vi "Set status to Idle.vi"(10 "Next state queue data":T1, 11 "UI queue":refnum<queue>) -> ()   [LabVIEW 2013]
uses:
  Typedefs/Next state queue data.ctl
  Typedefs/Start-Stop Enum.ctl
  Typedefs/Top level VI states.ctl
  Queue/Message Queue/Typedefs/Message Cluster.ctl
  Global Variables/General Globals.vi
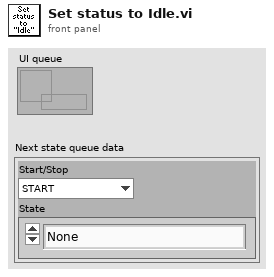
[diagram p1: front panel]
types:
  T1 = typedef "Next state queue data.ctl" = cluster{"Start/Stop":T2, "State":T3}
  T2 = typedef "Start-Stop Enum.ctl" = enum16{"START", "STOP"}
  T3 = typedef "Top level VI states.ctl" = enum16{"None", "Initialise UI", "<STACK PROTOCOL STATES>", "AOL Zstack-START", "AOL Zstack-STOP", "Motor Zstack-START", "Motor Zstack-STOP", "<ACQUISITION PROTOCOL STATES> ", "Functional Acquisition-START", "Functional Acquisition-STOP", "Single Plane Acquisition-START", "Single Plane Acquisition-STOP", "Volume Acquisition-START", "Volume Acquisition-STOP", "<LIVE IMAGING PROTOCOL STATES>", "Live Imaging-START", "Live Imaging-STOP", "Live Plane Imaging-START", "Live Plane Imaging-STOP", "Live Volume Imaging-START", "Live Volume Imaging-STOP", "EXIT"}
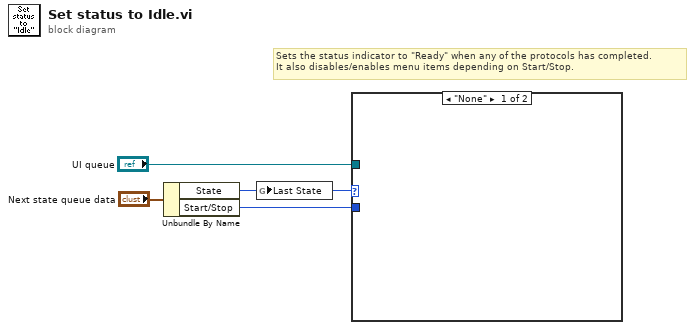
[diagram p0: block diagram]
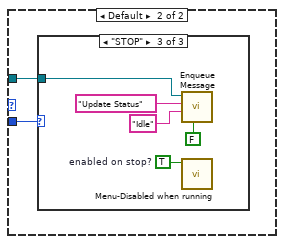
[diagram p2: hidden frame]
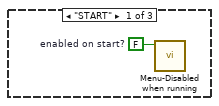
[diagram p3: hidden frame]
diagram:
  # "Sets the status indicator to \"Ready\" when any of the protocols has completed.\nIt also disables/enables menu items depending on Start/Stop."
  n1 = Unbundle By Name("Next state queue data") -> ("State"=w1:T3, "Start/Stop"=w3:T2)
  n2 = global write "General Globals.vi" "Last State"(w1) -> ()
  n3 = case shown="\"None\"" w1 {
    tunnel: w3 -> [_ w6]
    tunnel: "UI queue" -> [_ w5]
    frame "None" {
    }
    frame Default {
      n4 = case shown="\"STOP\"" w6 {
        tunnel: w5 -> [_ _ w8]
        frame "START" {
          w7 = FALSE  # enabled on start?
          n5 = call "Menu-Disabled when running.vi"("enabled?"=w7) -> ()  [unwired: 10 in, 1 out]
        }
        frame Default {
        }
        frame "STOP" {
          w12 = TRUE  # enabled on stop?
          n6 = call "Enqueue Message.vi"("Priority Message? (F)"=FALSE, "Message Data"="Idle" ("Message"), "Message"="Update Status", "Queue"=w8) -> ()  [unwired: 6 in, 2 out]
          n7 = call "Menu-Disabled when running.vi"("enabled?"=w12) -> ()  [unwired: 10 in, 1 out]
        }
      }
    }
  }
